vi "Get RefNum.vi"(8 "error in (no error)":errorcluster, 11 "Spectrometer iHR320 in":refnum<class "Spectrometer iHR320.lvclass">) -> (0 "error out":errorcluster, 2 "RefNum":refnum<k7>, 3 "Spectrometer iHR320 out":refnum<class "Spectrometer iHR320.lvclass">)   [LabVIEW 2009, in "Spectrometer iHR320.lvclass"]
doc: "Returns the active RefNum for the spectrometer."
uses:
  Spectrometer iHR320.lvclass
  Spectrometer iHR320.lvclass/Spectrometer iHR320.ctl
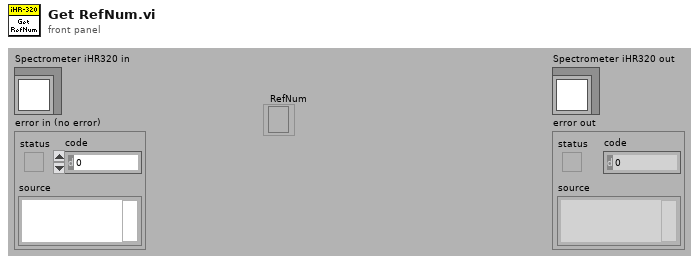
[diagram p1: front panel]
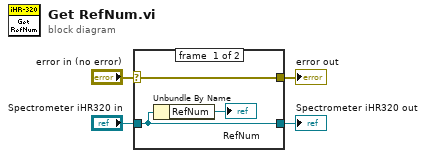
[diagram p0: block diagram]
diagram:
  n1 = case shown="No Error" "error in (no error)" {
    selector: "error in (no error)" -> [w6 w9]
    tunnel: [w6 w9] -> w3
    tunnel: [w5 w8] -> w2
    tunnel: "Spectrometer iHR320 in" -> [w5 w8]
    frame #0 {
      n2 = Unbundle By Name(w5) -> ("RefNum"=→"RefNum":refnum<k7>)
    }
    frame #1 {
    }
  }
  "Spectrometer iHR320 out" <- w2
  "error out" <- w3
